vi "MGCC_visualization_phasetwo_v2.vi"() -> ()   [LabVIEW 2016]
uses:
  Black start/Sub-VIs/MGCC_BlkStart_Globals.vi
  MGCC_FntStaMach_gobal.vi
  Resynchronization/MGCC_Resync_global.vi
  Communication/Global communication output.vi
  Communication/Global communication.vi
  <vilib>/imath/engines/lvmath2/RunTimeEngine/IndexRead/NIMS M($,S).vi
  <instcachedir>/0/NIMS M($,S)_3E5749BBB62E49528D4765A77F1F6D98.lvgen/NIMS M($,S)_3E5749BBB62E49528D4765A77F1F6D98_002.vi
  <vilib>/imath/engines/lvmath2/RunTimeEngine/BuiltInFunctions/length/NIMS_length(GV).vi
  <instcachedir>/0/NIMS_length(GV)_08A3D13377FD4E4B96F5795FBF3698FA.lvgen/NIMS_length(GV)_08A3D13377FD4E4B96F5795FBF3698FA_002.vi
  <vilib>/imathl/engines/lvmath/Functions/Error Handling/Create Error.vi
  <vilib>/imath/engines/lvmath2/RunTimeEngine/RangeToken/NIMS_Range_R3 - Integer.vi
  <instcachedir>/0/NIMS_Range_R3 - Integer_A435E2FF893B4C718FD5055FE39FE2F6.lvgen/NIMS_Range_R3 - Integer_A435E2FF893B4C718FD5055FE39FE2F6_000.vi
  <vilib>/imath/engines/lvmath2/RunTimeEngine/CommandStatement/MC_CommandStatement_break.vi
  <vilib>/imath/engines/lvmath2/RunTimeEngine/IndexReplace/NIMS M(S,S)=S.vi
  <instcachedir>/0/NIMS M(S,S)=S_98E40400474E4398B113AE20298B4F82.lvgen/NIMS M(S,S)=S_98E40400474E4398B113AE20298B4F82_002.vi
  <instcachedir>/0/NIMS M($,S)_3E5749BBB62E49528D4765A77F1F6D98.lvgen/NIMS M($,S)_3E5749BBB62E49528D4765A77F1F6D98_000.vi
  <instcachedir>/0/NIMS_length(GV)_08A3D13377FD4E4B96F5795FBF3698FA.lvgen/NIMS_length(GV)_08A3D13377FD4E4B96F5795FBF3698FA_000.vi
  <vilib>/imath/engines/lvmath2/RunTimeEngine/IndexRead/NIMS M(S,$).vi
  <instcachedir>/0/NIMS M(S,$)_F24F360562DE41D8BE234322A2E15C65.lvgen/NIMS M(S,$)_F24F360562DE41D8BE234322A2E15C65_000.vi
  <vilib>/imath/engines/lvmath2/RunTimeEngine/IndexRead/NIMS M(S,S).vi
  <instcachedir>/0/NIMS M(S,S)_AC51E74150A542F7991B9634C66F3096.lvgen/NIMS M(S,S)_AC51E74150A542F7991B9634C66F3096_000.vi
  <instcachedir>/0/NIMS M(S,S)=S_98E40400474E4398B113AE20298B4F82.lvgen/NIMS M(S,S)=S_98E40400474E4398B113AE20298B4F82_000.vi
  <vilib>/imath/engines/lvmath2/RunTimeEngine/BuiltInFunctions/is_empty/NIMS_is_empty(GM).vi
  <instcachedir>/0/NIMS_is_empty(GM)_AF8F13F4B7FD436CB1855477E2504B8A.lvgen/NIMS_is_empty(GM)_AF8F13F4B7FD436CB1855477E2504B8A_004.vi
  <vilib>/imath/engines/lvmath2/RunTimeEngine/IndexRead/NIMS M(R2,S).vi
  <instcachedir>/0/NIMS M(R2,S)_56813DCFDD5A484292D2195AF15D2BF5.lvgen/NIMS M(R2,S)_56813DCFDD5A484292D2195AF15D2BF5_000.vi
  <vilib>/imath/engines/lvmath2/RunTimeSupport/NIMS_Error if Not Equal.vi
  <instcachedir>/0/NIMS_Error if Not Equal_43252A79AD05436189442EC0C5E5AB8A.lvgen/NIMS_Error if Not Equal_43252A79AD05436189442EC0C5E5AB8A_000.vi
  <vilib>/imath/engines/lvmath2/RunTimeEngine/ErrorHandling/NIMS_Create Error From Enums.vi
  <vilib>/imath/engines/lvmath2/RunTimeEngine/NodeEndStatement/NIMS_NodeEndStatement_Output.vi
  <instcachedir>/0/NIMS_NodeEndStatement_Output_53EC0D466D134D7ABD903AC30B43404B.lvgen/NIMS_NodeEndStatement_Output_53EC0D466D134D7ABD903AC30B43404B_010.vi
  <vilib>/imath/engines/lvmath2/RunTimeEngine/ErrorHandling/NIMS_Finalize Error.vi
  <vilib>/imath/engines/lvmath2/RunTimeEngine/BuiltInFunctions/findnz/NIMS_[1o]_findnz(GRowV).vi
  <instcachedir>/0/NIMS_[1o]_findnz(GRowV)_1AF74843B4874134ADE908C0A4A72F3C.lvgen/NIMS_[1o]_findnz(GRowV)_1AF74843B4874134ADE908C0A4A72F3C_000.vi
  <vilib>/imath/engines/lvmath2/RunTimeEngine/BuiltInFunctions/is_empty/NIMS_is_empty(GV).vi
  <instcachedir>/0/NIMS_is_empty(GV)_FC7E7C3D9544432CB6AA2416ADCF6D56.lvgen/NIMS_is_empty(GV)_FC7E7C3D9544432CB6AA2416ADCF6D56_000.vi
  <vilib>/imath/engines/lvmath2/RunTimeEngine/IndexReplace/NIMS V(S)=S.vi
  <instcachedir>/0/NIMS V(S)=S_57E16554CB8B4B90AAB163894F717546.lvgen/NIMS V(S)=S_57E16554CB8B4B90AAB163894F717546_003.vi
  <vilib>/imath/engines/lvmath2/RunTimeEngine/IndexReplace/NIMS V(S)=V.vi
  <instcachedir>/0/NIMS V(S)=V_623363232DF04CF88CEE4AC156064DF2.lvgen/NIMS V(S)=V_623363232DF04CF88CEE4AC156064DF2_000.vi
  <instcachedir>/0/NIMS_NodeEndStatement_Output_53EC0D466D134D7ABD903AC30B43404B.lvgen/NIMS_NodeEndStatement_Output_53EC0D466D134D7ABD903AC30B43404B_004.vi
  <vilib>/imath/engines/lvmath2/RunTimeEngine/IndexRead/NIMS V(S).vi
  <instcachedir>/0/NIMS V(S)_0488751826AF41519A22953C041130DC.lvgen/NIMS V(S)_0488751826AF41519A22953C041130DC_000.vi
  <instcachedir>/0/NIMS V(S)=S_57E16554CB8B4B90AAB163894F717546.lvgen/NIMS V(S)=S_57E16554CB8B4B90AAB163894F717546_000.vi
  <instcachedir>/0/NIMS_NodeEndStatement_Output_53EC0D466D134D7ABD903AC30B43404B.lvgen/NIMS_NodeEndStatement_Output_53EC0D466D134D7ABD903AC30B43404B_005.vi
  State Estimation/Sub-VIs/MGCC_StaEst_global.vi
  Planned Islanding(Mark)/Sub VIs/MGCC_PlanISD_Global.vi
panel:
  in  "planned ISD 29":bool
  in  "planned ISD1":bool
  in  "LC2_reboot":bool
  in  "LC1_reboot":bool
  out "StaEst_An":dbl[][][](array[numeric])
  out "StaEst_Vn":dbl[][][](array[numeric])
  out "Overall MG states":string
  out "L13 line 3":u32(colorbox)
  out "?":bool
  in  "?":dbl(slide) scale=0.0..2.0
  out "LC1 state":string
  out "LC2 state":string
  in  "BKS cmd 2":bool=TRUE
  out "error out":errorcluster
  out "SW 2":u32(colorbox)
  out "G 1":u32(colorbox)
  out "L8":u32(colorbox)
  out "L7 line 2":u32(colorbox)
  out "L6 line 5":u32(colorbox)
  out "L6 line 1":u32(colorbox)
  out "SW 8":u32(colorbox)
  out "SW 8 off":u32(colorbox)
  out "I 8":dbl format="%#.4f"
  out "L6":u32(colorbox)
  out "Communication":bool
  out "Resynchronization":bool
  out "Active power control":bool
  out "Reactive power control":bool
  out "SOC1":dbl=0.5979085480424442 format="%#_4f"
  out "Output":dbl=-9.999999999999723e-06 format="%#_4f"
  in  "PV Mode":bool
  out "Output 3":dbl=0.40429047942961227 format="%#_4f"
  out "Communication 2":bool
  out "Resynchronization 2":bool
  out "Active power control 2":bool
  out "Reactive power control 2":bool
  out "SOC 2":dbl=0.5 format="%#_4f"
  out "Output 2":dbl format="%#_4f"
  out "SW 6":u32(colorbox)
  out "SW 6 off":u32(colorbox)
  out "SW 7":u32(colorbox)
  out "SW 7 off":u32(colorbox)
  out "SW 4":u32(colorbox)
  out "SW 4 off":u32(colorbox)
  out "SW 5":u32(colorbox)
  out "SW 5 off":u32(colorbox)
  out "SW 1":u32(colorbox)
  out "SW 1 off":u32(colorbox)
  out "SW 2 off":u32(colorbox)
  out "SW 3":u32(colorbox)
  out "SW 3 off":u32(colorbox)
  out "I 7":dbl format="%#.4f"
  out "I 3":dbl format="%#.4f"
  out "I 4":dbl format="%#.4f"
  out "I 2":dbl format="%#.4f"
  out "I 6":dbl format="%#.4f"
  out "I 5":dbl format="%#.4f"
  out "I 1":dbl format="%#.4f"
  out "Model Mgmt.":bool
  out "PV Forecasting":bool
  out "Load Forecasting":bool
  out "PQ Balance":bool
  out "Black Start":bool
  out "Data Logging":bool
  out "Communication":bool
  out "State Estimation":bool
  out "Energy Mgmt.":bool
  out "G1 state":string
  in  "Stop":bool
  in  "RESET":bool
  in  "G1":bool
  in  "Ready for STD":bool
  in  "Recon cmd":bool
  in  "BKS cmd":bool=TRUE
  in  "Power Tabs":T1(tab)
  out "Loads Power 6":dbl(graph)
  out "Loads Power 7":dbl(graph)
  out "Loads Power 8":dbl(graph)
  out "Loads Power 9":dbl(graph)
  out "Loads Power 10":dbl(graph)
  out "Loads Power 11":dbl(graph)
  out "Loads Power 12":dbl(graph)
  out "Loads Power 13":dbl(graph)
  in  "Voltage Tabs":T1(tab)
  out "Voltage 6":dbl(graph)
  out "Voltage 7":dbl(graph)
  out "Voltage 8":dbl(graph)
  out "Voltage 9":dbl(graph)
  out "Voltage 10":dbl(graph)
  out "Voltage 11":dbl(graph)
  out "Voltage 12":dbl(graph)
  out "Voltage 13":dbl(graph)
  out "Frequency":T2(graph)
  out "Sources Power":T3(graph)
  out "L11 line 2":u32(colorbox)
  out "L11 line 1":u32(colorbox)
  out "L10 line 2":u32(colorbox)
  out "L12 line 2":u32(colorbox)
  out "G1 line 1":u32(colorbox)
  out "L8 line 2":u32(colorbox)
  out "L8 line 1":u32(colorbox)
  out "L13 line 1":u32(colorbox)
  out "PV line 1":u32(colorbox)
  out "B1 line 1":u32(colorbox)
  out "L13 line 2":u32(colorbox)
  out "B2":bool
  out "SOC Tank 2":dbl(slide) scale=0.0..1.0
  out "PV1":bool
  out "B1":bool
  out "SOC Tank1":dbl(slide) scale=0.0..1.0
  out "PV1 irr Tank":dbl(slide) scale=0.0..2.0
  out "L9 line1":u32(colorbox)
  out "B2 line 1":u32(colorbox)
  out "L9 line 2":u32(colorbox)
  out "L6 line 4":u32(colorbox)
  out "L9":u32(colorbox)
  out "L7":u32(colorbox)
  out "L7 line 1":u32(colorbox)
  out "L8 line 3":u32(colorbox)
  out "L13":u32(colorbox)
  out "L12":u32(colorbox)
  out "L12 line 1":u32(colorbox)
  out "L10 line 1":u32(colorbox)
  out "L11":u32(colorbox)
  out "L10":u32(colorbox)
  out "L6 line 2":u32(colorbox)
  out "L6 line 3":u32(colorbox)
  out "L8 line 4":u32(colorbox)
  out "Gen4 Tank 2":dbl(slide) scale=0.0..1.0
  # "Opal-RT HIL Test Bed Controller"
  # "G5"
  # "SW8"
  # "SW5"
  # "SW1"
  # "SW6"
  # "L6"
  # "L10"
  # "L11"
  # "Local Controller 1"
  # "PV"
  # "BESS1 & PV"
  # "SW2"
  # "SW4"
  # "L7"
  # "L12"
  # "-Manual"
  # "-Profile"
  # "SW7"
  # "SW3"
  # "Local Controller 2"
  # "L8"
  # "Central Controller"
  # "L9"
  # "L13"
  # "BESS2"
  # "Gen4"
  # "BESS1"
  # "PV3"
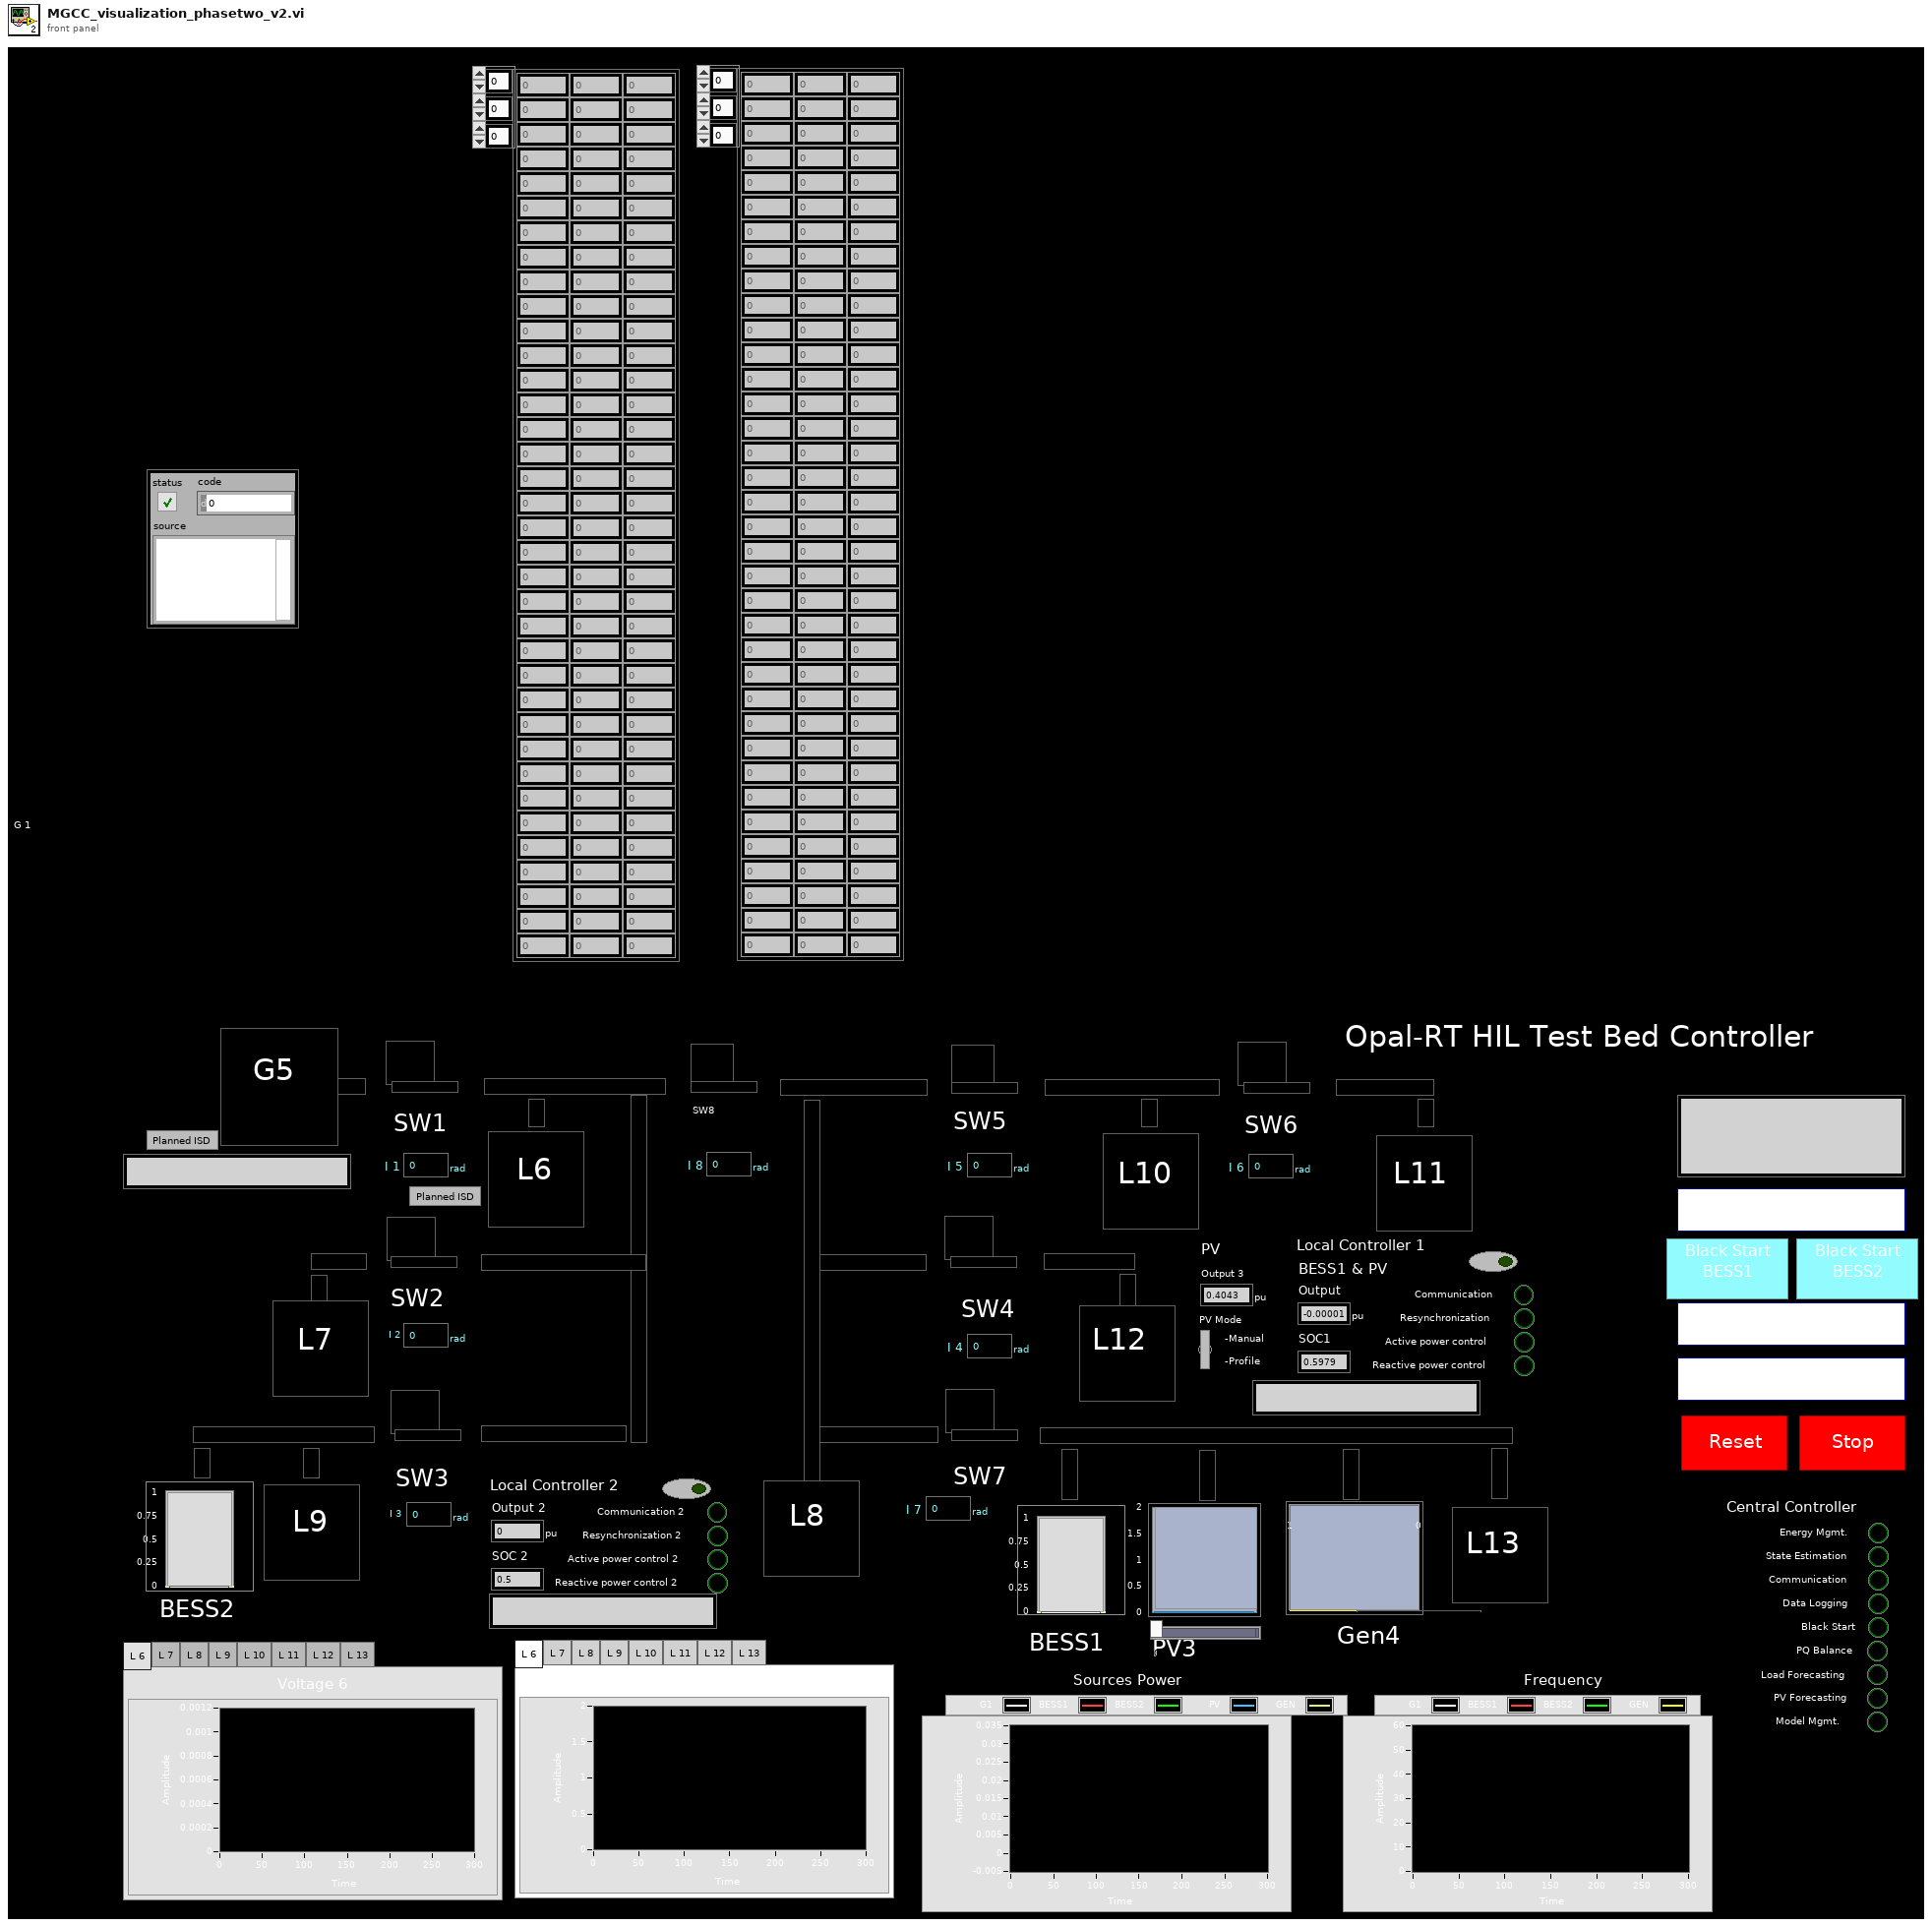
[diagram p1: front panel]
types:
  T1 = enum32{"L 6", "L 7", "L 8", "L 9", "L 10", "L 11", "L 12", "L 13"}
  T2 = cluster{"Numeric":dbl, "Numeric":dbl, "Numeric":dbl, "Numeric 2":dbl}
  T3 = cluster{"Numeric":dbl, "Numeric":dbl, "Numeric":dbl, "Numeric":dbl, "Numeric":dbl}
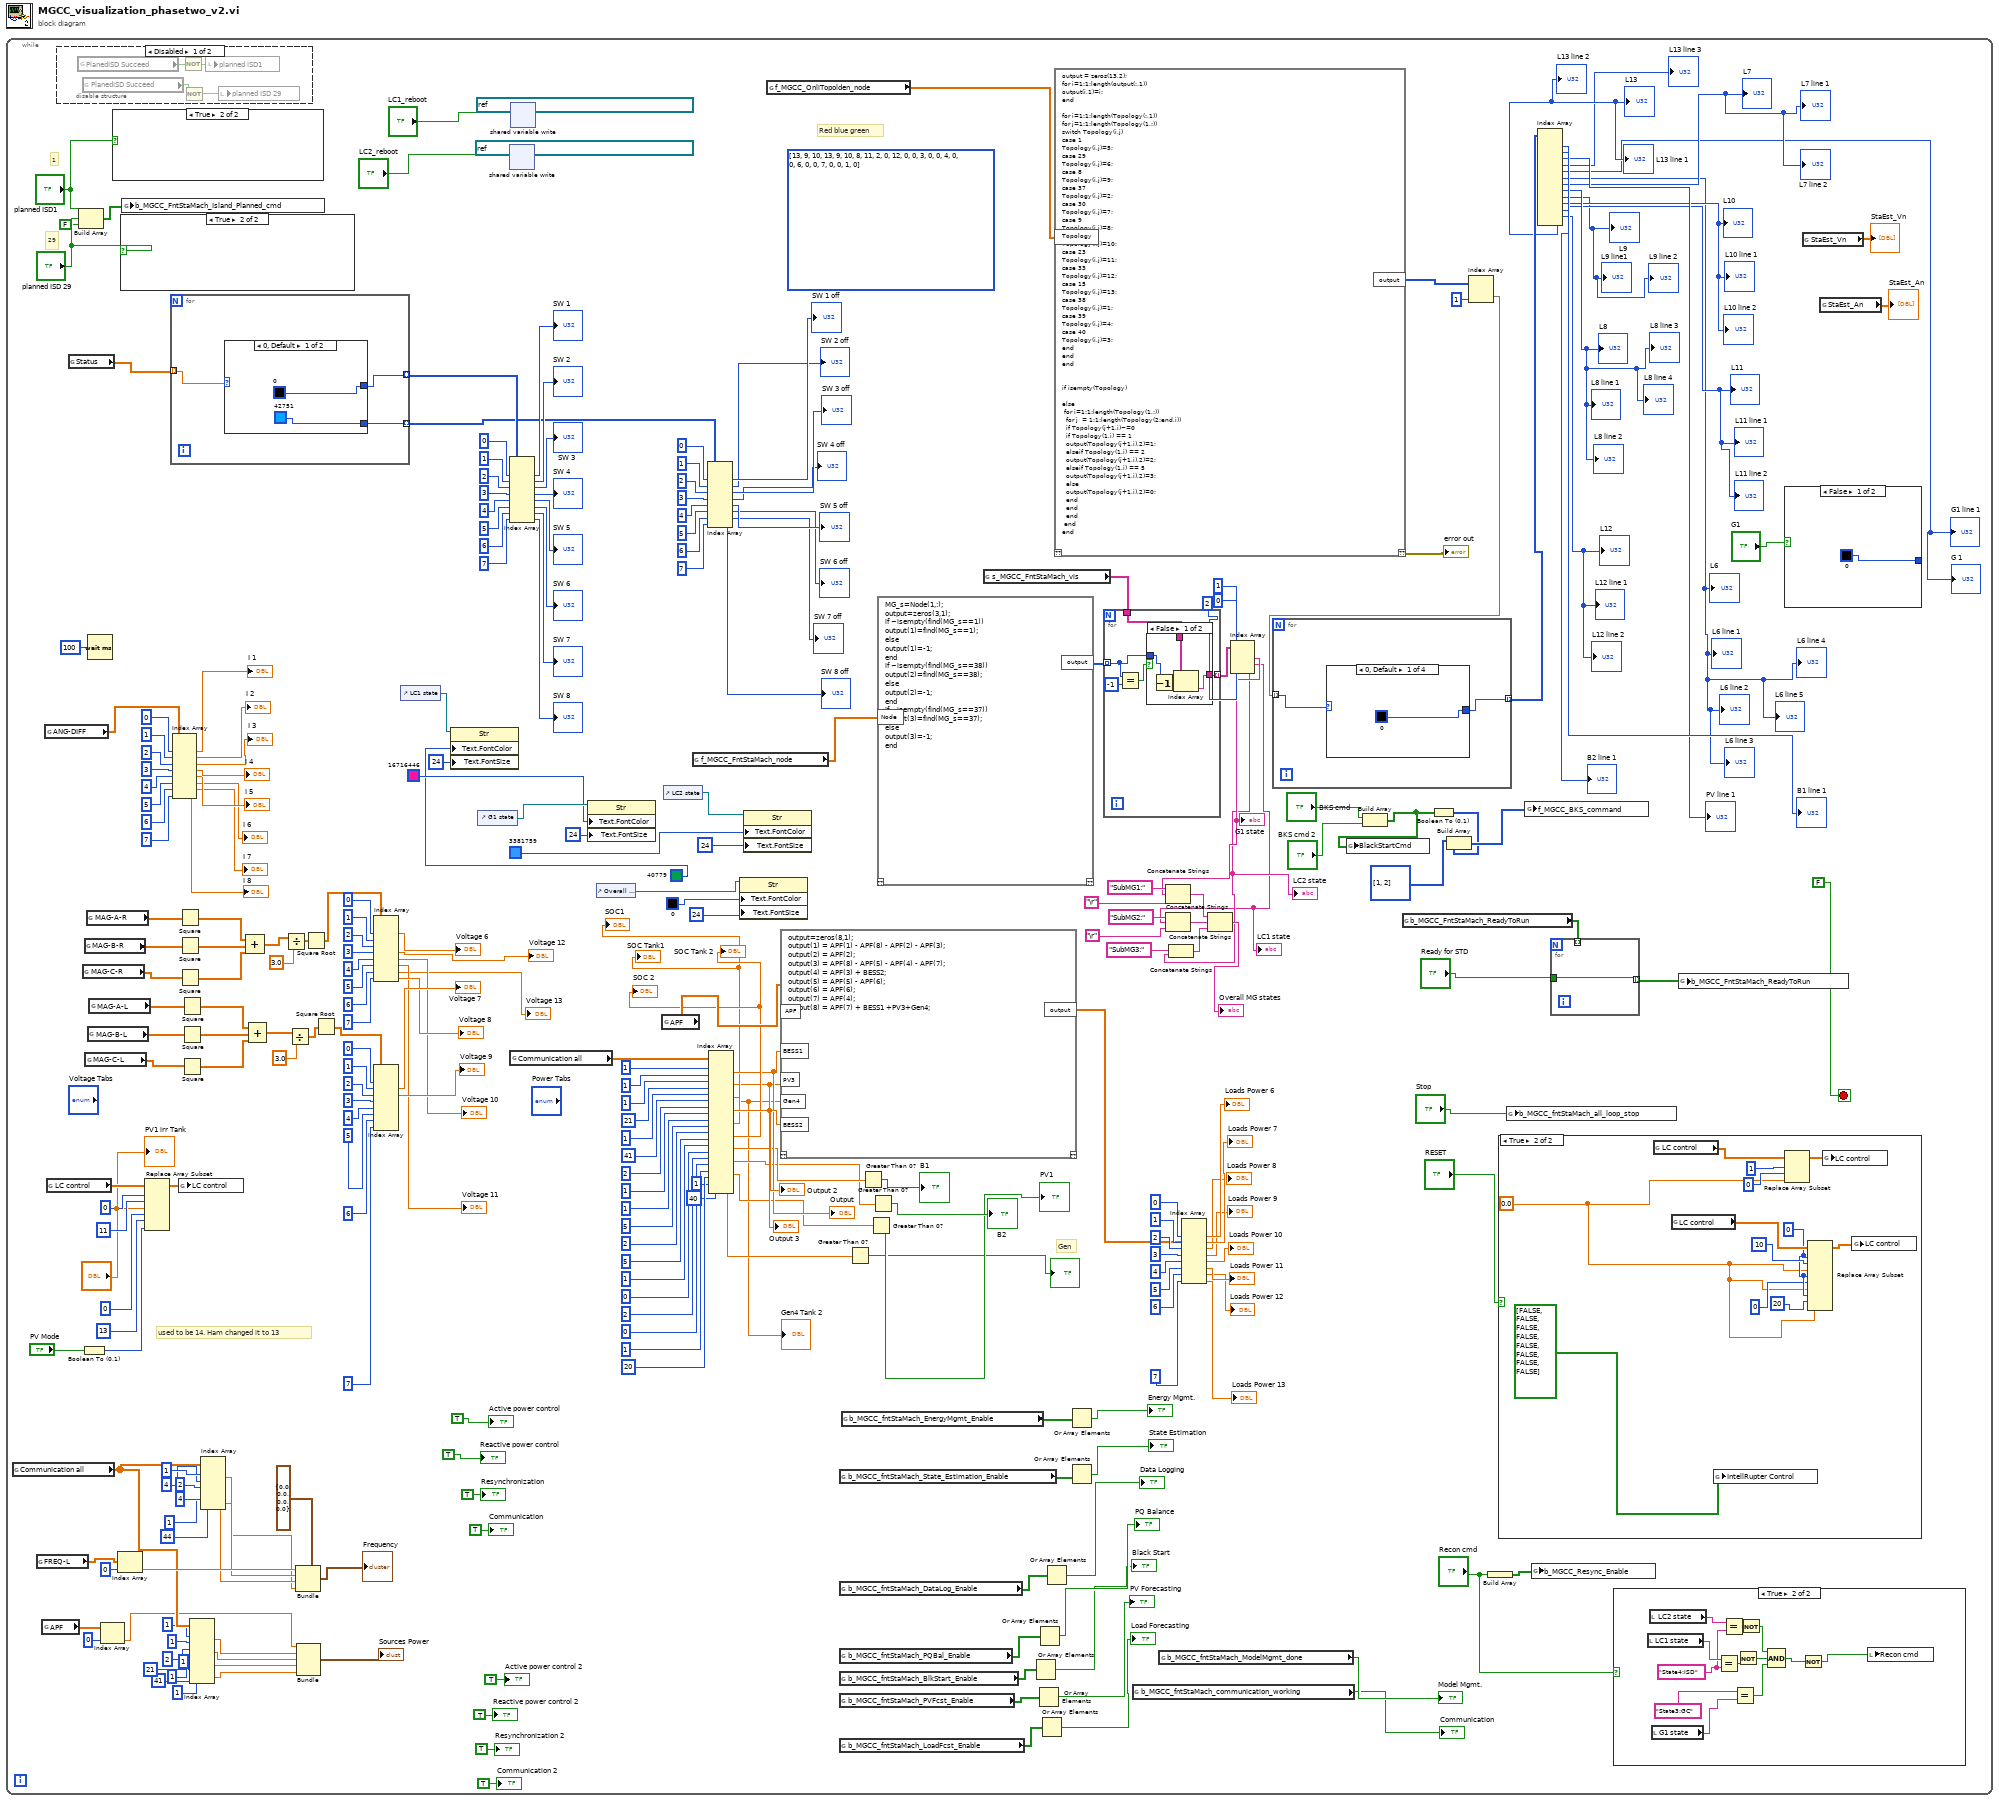
[diagram p0: block diagram]
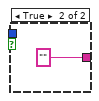
[diagram p7: hidden frame]
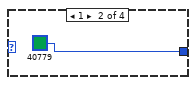
[diagram p8: hidden frame]
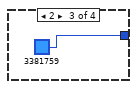
[diagram p9: hidden frame]
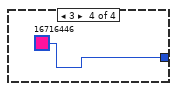
[diagram p10: hidden frame]
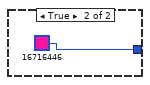
[diagram p11: hidden frame]
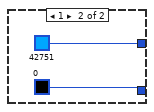
[diagram p12: hidden frame]
diagram:
  n1 = while {
    stop <- FALSE stop-if-true
    (unwired) i32[][] [[13, 9, 10], [13, 9, 10], [8, 11, 2], [0, 12, 0], [0, 3, 0], [0, 4, 0], [0, 6, 0], [0, 7, 0], [0, 1, 0]]
    # "1"
    # "29"
    # "used to be 14. Ham changed it to 13"
    # "Gen"
    # "Red blue green"
    # "9 10: bESS\n11 12: PV gen\n13: g1\n1 to 8: load"
    n2 = global read "Global communication.vi" "Communication all"() -> (w94:dbl[][])
    n3 = global read "Global communication.vi" "FREQ-L"() -> (w99:dbl[])
    n4 = global read "Global communication.vi" "APF"() -> (w87:dbl[])
    n5 = global read "Global communication.vi" "ANG-DIFF"() -> (w206:dbl[])
    n6 = global read "Global communication.vi" "LC control"() -> (w116:dbl[][])
    n7 = disable-structure shown="Disabled" {
      frame Disabled {
        n8 = global read "MGCC_PlanISD_Global.vi" "PlanedISD Succeed"() -> (w292:bool)
        n9 = global read "MGCC_PlanISD_Global.vi" "PlanedISD Succeed"() -> (w290:bool)
        n10 = Not(x=w292) -> (.not. x?=w293:bool)
        n11 = Not(x=w290) -> (.not. x?=w291:bool)
        n12 = local write "planned ISD1"(w293) -> ()
        n13 = local write "planned ISD 29"(w291) -> ()
      }
      frame Enabled {
      }
    }
    n14 = global read "Global communication.vi" "Status"() -> (w289:dbl[])
    n15 = Build Array("planned ISD1", "planned ISD 29", FALSE ("element")) -> (w4:bool[])
    n16 = Boolean To (0,1)(Boolean="PV Mode") -> (0, 1=w104:i16)
    n17 = global read "Global communication.vi" "MAG-C-R"() -> (w189:dbl[])
    n18 = global read "Global communication.vi" "MAG-B-R"() -> (w190:dbl[])
    n19 = global read "Global communication.vi" "MAG-C-L"() -> (w195:dbl[])
    n20 = global read "Global communication.vi" "MAG-A-R"() -> (w191:dbl[])
    n21 = Wait (ms)(milliseconds to wait=u32 100) -> ()  [unwired: 1 out]
    n22 = global read "Global communication.vi" "MAG-B-L"() -> (w196:dbl[])
    n23 = global read "Global communication.vi" "MAG-A-L"() -> (w197:dbl[])
    n24 = Index Array(array=w87, index=0) -> (element=w85:dbl)
    n25 = case shown="True" "planned ISD1" {
      frame False {
      }
      frame True {
      }
    }
    n26 = Index Array(array=w99, index=0) -> (element=w97:dbl)
    n27 = case shown="True" "planned ISD 29" {
      frame False {
      }
      frame True {
      }
    }
    n28 = global write "MGCC_FntStaMach_gobal.vi" "b_MGCC_FntStaMach_Island_Planned_cmd"(w4) -> ()
    n29 = Replace Array Subset(array=w116, new element #1="?", index (row) #1=0 ("index (row)"), index (col) #1=11 ("disabled index (col)"), new element #2=w104, index (row) #2=0 ("index (row)"), index (col) #2=13 ("disabled index (col)")) -> (w115:dbl[][])
    n30 = for {
      tunnel: w289 -> [w2198] mode=indexing
      tunnel: [w2197] -> w288 mode=indexing
      tunnel: [w2196] -> w263 mode=indexing
      n31 = case shown="0, Default" w2198 {
        tunnel: [u32 0 ("Color Box 17") u32 42751 ("Color Box 17")] -> w2197
        tunnel: [u32 42751 ("Color Box 17") u32 0 ("Color Box 17")] -> w2196
        frame 0, Default {
        }
        frame 1 {
        }
      }
    }
    n32 = Index Array(array=w206, index #1=0 ("index"), index #2=1 ("index"), index #3=2 ("index"), index #4=3 ("index"), index #5=4 ("index"), index #6=5 ("index"), index #7=6 ("index"), index #8=7 ("index")) -> (element #1=→"I 1":dbl, element #2=→"I 2":dbl, element #3=→"I 3":dbl, element #4=→"I 4":dbl, element #5=→"I 5":dbl, element #6=→"I 6":dbl, element #7=→"I 7":dbl, element #8=→"I 8":dbl)
    n33 = Square(x=w191) -> (x^2=w188:dbl[])
    n34 = Square(x=w190) -> (x^2=w187:dbl[])
    n35 = Square(x=w189) -> (x^2=w186:dbl[])
    n36 = global write "Global communication.vi" "LC control"(w115) -> ()
    n37 = Square(x=w197) -> (x^2=w194:dbl[])
    n38 = Square(x=w196) -> (x^2=w193:dbl[])
    n39 = Square(x=w195) -> (x^2=w192:dbl[])
    n40 = Index Array(array=w94, index (row) #1=1 ("index (row)"), index (col) #1=1 ("disabled index (col)"), index (row) #2=2 ("index (row)"), index (col) #2=1 ("disabled index (col)"), index (row) #3=1 ("index (row)"), index (col) #3=21 ("disabled index (col)"), index (row) #4=1 ("index (row)"), index (col) #4=41 ("disabled index (col)")) -> (element #1=w89:dbl, element #2=w88:dbl, element #3=w18:dbl, element #4=w17:dbl)
    n41 = Index Array(array=w94, index (row) #1=1 ("index (row)"), index (col) #1=4 ("disabled index (col)"), index (row) #2=2 ("index (row)"), index (col) #2=4 ("disabled index (col)"), index (row) #3=1 ("index (row)"), index (col) #3=44 ("disabled index (col)")) -> (element #1=w96:dbl, element #2=w95:dbl, element #3=w14:dbl)
    n42 = Compound Arithmetic op=ADD(w188, w187, w186) -> (w11:dbl[])
    n43 = Compound Arithmetic op=ADD(w194, w193, w192) -> (w8:dbl[])
    n44 = Divide(x=w11, y=3.0) -> (x/y=w12:dbl[])
    n45 = Divide(x=w8, y=3.0) -> (x/y=w7:dbl[])
    n46 = Bundle(cluster=T2 {"Numeric"=0.0, "Numeric"=0.0, "Numeric"=0.0, "Numeric 2"=0.0}, "Numeric"=w97, "Numeric"=w96, "Numeric"=w95, "Numeric 2"=w14) -> (→"Frequency":T2)
    n47 = Bundle("Numeric"=w85, "Numeric"=w89, "Numeric"=w88, "Numeric"=w18, "Numeric"=w17) -> (→"Sources Power":T3)  [unwired: 1 in]
    n48 = Square Root(x=w12) -> (sqrt(x)=w169:dbl[])
    n49 = Square Root(x=w7) -> (sqrt(x)=w168:dbl[])
    n50 = Index Array(array=w169, index #1=0 ("index"), index #2=1 ("index"), index #3=2 ("index"), index #4=3 ("index"), index #5=4 ("index"), index #6=5 ("index"), index #7=6 ("index"), index #8=7 ("index")) -> (element #1=→"Voltage 6":dbl, element #4=→"Voltage 12":dbl, element #5=→"Voltage 10":dbl, element #6=→"Voltage 11":dbl, element #7=→"Voltage 13":dbl, element #8=→"Voltage 8":dbl)  [unwired: 2 out]
    n51 = Index Array(array=w168, index #1=0 ("index"), index #2=1 ("index"), index #3=2 ("index"), index #4=3 ("index"), index #5=4 ("index"), index #6=5 ("index"), index #7=6 ("index"), index #8=7 ("index")) -> (element #2=→"Voltage 7":dbl, element #3=→"Voltage 9":dbl)  [unwired: 6 out]
    n52 = control-ref of="LC1 state"() -> (w219:refnum<vi>)
    n53 = property on="Property Node" class="Str"(reference=w219, "Text.FontColor"=u32 40779 ("Color Box 17"), "Text.FontSize"=u32 24 ("Text.Font:Size")) -> ()  [unwired: 1 in, 2 out]
    n54 = control-ref of="G1 state"() -> (w223:refnum<vi>)
    n55 = shared-variable-write(refnum<k21> "ni.var.psp://LC2/Untitled Library 2/LC2_reboot" ("shared variable refnum in"), "LC2_reboot") -> ()  [unwired: 1 in, 2 out]
    n56 = Index Array(array=w288, index #1=0 ("index"), index #2=1 ("index"), index #3=2 ("index"), index #4=3 ("index"), index #5=4 ("index"), index #6=5 ("index"), index #7=6 ("index"), index #8=7 ("index")) -> (element #1=→"SW 1":u32, element #2=→"SW 2":u32, element #3=→"SW 3":u32, element #4=→"SW 4":u32, element #5=→"SW 5":u32, element #6=→"SW 6":u32, element #7=→"SW 7":u32, element #8=→"SW 8":u32)
    n57 = global read "Global communication.vi" "Communication all"() -> (w141:dbl[][])
    n58 = shared-variable-write(refnum<k21> "ni.var.psp://LC1/Untitled Library 1/LC1_reboot" ("shared variable refnum in"), "LC1_reboot") -> ()  [unwired: 1 in, 2 out]
    n59 = property on="Property Node" class="Str"(reference=w223, "Text.FontColor"=u32 16716446 ("Color Box 17"), "Text.FontSize"=u32 24 ("Text.Font:Size")) -> ()  [unwired: 1 in, 2 out]
    n60 = control-ref of="Overall MG states"() -> (w29:refnum<vi>)
    n61 = global read "Global communication.vi" "APF"() -> (w159:dbl[])
    n62 = control-ref of="LC2 state"() -> (w218:refnum<vi>)
    n63 = global read "MGCC_FntStaMach_gobal.vi" "f_MGCC_FntStaMach_node"() -> (w230:dbl[])
    n64 = Index Array(array=w263, index #1=0 ("index"), index #2=1 ("index"), index #3=2 ("index"), index #4=3 ("index"), index #5=4 ("index"), index #6=5 ("index"), index #7=6 ("index"), index #8=7 ("index")) -> (element #1=→"SW 1 off":u32, element #2=→"SW 2 off":u32, element #3=→"SW 3 off":u32, element #4=→"SW 4 off":u32, element #5=→"SW 5 off":u32, element #6=→"SW 6 off":u32, element #7=→"SW 7 off":u32, element #8=→"SW 8 off":u32)
    n65 = Index Array(array=w141, index (row) #1=1 ("index (row)"), index (col) #1=1 ("disabled index (col)"), index (row) #2=1 ("index (row)"), index (col) #2=21 ("disabled index (col)"), index (row) #3=1 ("index (row)"), index (col) #3=41 ("disabled index (col)"), index (row) #4=2 ("index (row)"), index (col) #4=1 ("disabled index (col)"), index (row) #5=1 ("index (row)"), index (col) #5=5 ("disabled index (col)"), index (row) #6=2 ("index (row)"), index (col) #6=5 ("disabled index (col)"), index (row) #7=1 ("index (row)"), index (col) #7=0 ("disabled index (col)"), index (row) #8=2 ("index (row)"), index (col) #8=0 ("disabled index (col)"), index (row) #9=1 ("index (row)"), index (col) #9=20 ("disabled index (col)"), index (row) #10=1 ("index (row)"), index (col) #10=40 ("disabled index (col)")) -> (element #1=w127:dbl, element #2=w125:dbl, element #3=w42:dbl, element #4=w129:dbl, element #5=→"SOC Tank1" →"SOC1":dbl, element #6=→"SOC 2" →"SOC Tank 2":dbl, element #7=w120:dbl, element #8=w118:dbl, element #9=w109:dbl, element #10=w45:dbl)
    "Output 2" <- w129
    "Output" <- w127
    "Output 3" <- w125
    "Gen4 Tank 2" <- w42
    n66 = property on="Property Node" class="Str"(reference=w29, "Text.FontColor"=u32 0 ("Color Box 17"), "Text.FontSize"=u32 24 ("Text.Font:Size")) -> ()  [unwired: 1 in, 2 out]
    n67 = property on="Property Node" class="Str"(reference=w218, "Text.FontColor"=u32 3381759 ("Color Box 17"), "Text.FontSize"=u32 24 ("Text.Font:Size")) -> ()  [unwired: 1 in, 2 out]
    n68 = global read "MGCC_FntStaMach_gobal.vi" "f_MGCC_OnliTopolden_node"() -> (w246:dbl[][])
    n69 = mathscript code="output=zeros(8,1);\noutput(1) = APF(1) - APF(8) - APF(2) - APF(3);\noutput(2) = APF(2);\noutput(3) = APF(8) - APF(5) - APF(4) - APF(7);\noutput(4) = APF(3) + BESS2;\noutput(5) = APF(5) - APF(6);\noutput(6) = APF(6);\noutput(7) = APF(4);\noutput(8) = APF(7) + BESS1 +PV3+Gen4;"("APF"=w159, "BESS1"=w127, "PV3"=w125, "Gen4"=w42, "BESS2"=w129) -> ("output"=w150:dbl[])  [unwired: 1 in, 1 out]
    n70 = global read "MGCC_FntStaMach_gobal.vi" "b_MGCC_fntStaMach_State_Estimation_Enable"() -> (w73:bool[])
    n71 = global read "MGCC_FntStaMach_gobal.vi" "b_MGCC_fntStaMach_DataLog_Enable"() -> (w71:bool[])
    n72 = global read "MGCC_FntStaMach_gobal.vi" "b_MGCC_fntStaMach_PQBal_Enable"() -> (w69:bool[])
    n73 = global read "MGCC_FntStaMach_gobal.vi" "b_MGCC_fntStaMach_BlkStart_Enable"() -> (w67:bool[])
    n74 = global read "MGCC_FntStaMach_gobal.vi" "b_MGCC_fntStaMach_PVFcst_Enable"() -> (w65:bool[])
    n75 = global read "MGCC_FntStaMach_gobal.vi" "b_MGCC_fntStaMach_LoadFcst_Enable"() -> (w63:bool[])
    n76 = global read "MGCC_FntStaMach_gobal.vi" "b_MGCC_fntStaMach_EnergyMgmt_Enable"() -> (w75:bool[])
    n77 = Greater Than 0?(x=w45) -> (x > 0?=→"?":bool)
    n78 = Greater Than 0?(x=w120) -> (x > 0?=→"B1":bool)
    n79 = Greater Than 0?(x=w109) -> (x > 0?=→"PV1":bool)
    n80 = Greater Than 0?(x=w118) -> (x > 0?=→"B2":bool)
    n81 = mathscript code="MG_s=Node(1,:);\noutput=zeros(3,1);\nif ~isempty(find(MG_s==1))\noutput(1)=find(MG_s==1);\nelse\noutput(1)=-1;\nend\nif ~isempty(find(MG_s==38))\noutput(2)=find(MG_s==38);\nelse\noutput(2)=-1;\nend\nif ~isempty(find(MG_s==37))\noutput(3)=find(MG_s==37);\nelse\noutput(3)=-1;\nend"("Node"=w230) -> ("output"=w229:i32[])  [unwired: 1 in, 1 out]
    n82 = global read "MGCC_FntStaMach_gobal.vi" "s_MGCC_FntStaMach_vis"() -> (w228:string[])
    n83 = Or Array Elements(Boolean array=w67) -> (logical OR=→"Black Start":bool)
    n84 = Or Array Elements(Boolean array=w65) -> (logical OR=→"PV Forecasting":bool)
    n85 = Or Array Elements(Boolean array=w69) -> (logical OR=→"PQ Balance":bool)
    n86 = Or Array Elements(Boolean array=w63) -> (logical OR=→"Load Forecasting":bool)
    n87 = Or Array Elements(Boolean array=w71) -> (logical OR=→"Data Logging":bool)
    n88 = mathscript code="output = zeros(13,2);\nfor i=1:1:length(output(:,1))\noutput(i,1)=i;\nend\n\nfor i=1:1:length(Topology(:,1))\nfor j=1:1:length(Topology(1,:))\nswitch Topology(i,j)\ncase 1\nTopology(i,j)=5;\ncase 29\nTopology(i,j)=6;\ncase 8\nTopology(i,j)=9;\ncase 37\nTopology(i,j)=2;\ncase 30\nTopology(i,j)=7;\ncase 9\nTopology(i,j)=8;\ncase 35\nTopology(i,j)=10;\ncase 23\nTopology(i,j)=11;\ncase 33\nTopology(i,j)=12;\ncase 15\nTopology(i,j)=13;\ncase 38\nTopology(i,j)=1;\ncase 39\nTopology(i,j)=4;\ncase 40\nTopology(i,j)=3;\nend\nend\nend\n\n\nif isempty(Topology)\n\nelse\n for i=1:1:length(Topology(1,:))\n  for j  = 1:1:length(Topology(2:end,i))\n  if Topology(j+1,i)~=0\n  if Topology(1,i) == 1\n  output(Topology(j+1,i),2)=1;\n  elseif Topology(1,i) == 2\n  output(Topology(j+1,i),2)=2;\n  elseif Topology(1,i) == 5\n  output(Topology(j+1,i),2)=3;\n  else\n  output(Topology(j+1,i),2)=0;\n  end\n  end\n  end\n end\nend"("Topology"=w246) -> ("??"=→"error out":errorcluster, "output"=w251:i32[][])  [unwired: 1 in]
    n89 = Or Array Elements(Boolean array=w75) -> (logical OR=→"Energy Mgmt.":bool)
    n90 = Or Array Elements(Boolean array=w73) -> (logical OR=→"State Estimation":bool)
    n91 = for {
      tunnel: w229 -> [w596] mode=indexing
      tunnel: w228 -> [w595]
      tunnel: [w594] -> w227 mode=indexing
      n92 = Equal?(x=w596, y=-1) -> (x = y?=w597:bool)
      n93 = case shown="False" w597 {
        tunnel: [w599 ""] -> w594
        tunnel: w596 -> [w601 _]
        tunnel: w595 -> [w600 _]
        frame False {
          n94 = Decrement(x=w601) -> (x-1=w602:i32)
          n95 = Index Array(array=w600, index=w602) -> (element=w599:string)
        }
        frame True {
        }
      }
    }
    n96 = global read "MGCC_FntStaMach_gobal.vi" "b_MGCC_fntStaMach_communication_working"() -> (→"Communication":bool)
    n97 = global read "MGCC_FntStaMach_gobal.vi" "b_MGCC_fntStaMach_ModelMgmt_done"() -> (→"Model Mgmt.":bool)
    n98 = Index Array(array=w150, index #1=0 ("index"), index #2=1 ("index"), index #3=2 ("index"), index #4=3 ("index"), index #5=4 ("index"), index #6=5 ("index"), index #7=6 ("index"), index #8=7 ("index")) -> (element #1=→"Loads Power 6":dbl, element #2=→"Loads Power 7":dbl, element #3=→"Loads Power 8":dbl, element #4=→"Loads Power 9":dbl, element #5=→"Loads Power 10":dbl, element #6=→"Loads Power 11":dbl, element #7=→"Loads Power 12":dbl, element #8=→"Loads Power 13":dbl)
    n99 = Index Array(array=w227, index #1=0 ("index"), index #2=1 ("index"), index #3=2 ("index")) -> (element #1=w40:string, element #2=w19:string, element #3=w20:string)
    "LC2 state" <- w20
    "LC1 state" <- w19
    "G1 state" <- w40
    n100 = Concatenate Strings("SubMG1:", w40, "\r") -> (w35:string)
    n101 = Concatenate Strings("SubMG2:", w19, "\r") -> (w34:string)
    n102 = Concatenate Strings("SubMG3:", w20) -> (w33:string)
    n103 = Concatenate Strings(w35, w34, w33) -> (→"Overall MG states":string)
    n104 = Build Array("BKS cmd", "BKS cmd 2") -> (w13:bool[])
    n105 = global write "MGCC_BlkStart_Globals.vi" "BlackStartCmd"(w13) -> ()
    n106 = global read "MGCC_FntStaMach_gobal.vi" "b_MGCC_FntStaMach_ReadyToRun"() -> (w59:bool[])
    n107 = Boolean To (0,1)(Boolean=w13) -> (0, 1=w234:i16[])
    n108 = Build Array(i32[] [1, 2], w234) -> (w235:i32[][])
    n109 = Index Array(array=w251, index (col)=1 ("disabled index (col)")) -> (element=w249:i32[])  [unwired: 1 in]
    n110 = for {
      tunnel: w249 -> [w827] mode=indexing
      tunnel: [w826] -> w248 mode=indexing
      n111 = case shown="0, Default" w827 {
        tunnel: [u32 0 ("Color Box 17") u32 40779 ("Color Box 17") u32 3381759 ("Color Box 17") u32 16716446 ("Color Box 17")] -> w826
        frame 0, Default {
        }
        frame 1 {
        }
        frame 2 {
        }
        frame 3 {
        }
      }
    }
    n112 = Build Array("Recon cmd") -> (w6:bool[])
    n113 = case shown="True" "RESET" {
      frame False {
      }
      frame True {
        w307 = 0.0 ("new element/subarray")
        w310 = 0 ("index")
        n114 = global read "Global communication.vi" "LC control"() -> (w316:dbl[][])
        n115 = global read "Global communication.vi" "LC control"() -> (w314:dbl[][])
        n116 = global write "Global communication output.vi" "IntellRupter Control"(bool[] [FALSE, FALSE, FALSE, FALSE, FALSE, FALSE, FALSE, FALSE] ("IntellRupter Control")) -> ()
        n117 = Replace Array Subset(array=w316, new element=w307, index (row)=1 ("index"), index (col)=0 ("index")) -> (w315:dbl[][])
        n118 = Replace Array Subset(array=w314, new element #1=w307, index (row) #1=w310, index (col) #1=10 ("index"), new element #2=w307, index (row) #2=w310, index (col) #2=0 ("index"), new element #3=w307, index (row) #3=w310, index (col) #3=20 ("index")) -> (w313:dbl[][])
        n119 = global write "Global communication.vi" "LC control"(w315) -> ()
        n120 = global write "Global communication.vi" "LC control"(w313) -> ()
      }
    }
    n121 = global write "MGCC_FntStaMach_gobal.vi" "b_MGCC_fntStaMach_all_loop_stop"("Stop") -> ()
    n122 = global write "MGCC_FntStaMach_gobal.vi" "f_MGCC_BKS_command"(w235) -> ()
    n123 = global write "MGCC_Resync_global.vi" "b_MGCC_Resync_Enable"(w6) -> ()
    n124 = Index Array(array=w248) -> (element #1=→"B1 line 1":u32, element #2=→"B2 line 1":u32, element #3=→"PV line 1":u32, element #4=→"L13 line 3":u32, element #5=→"G1 line 1" →"G 1":u32, element #6=→"L6" →"L6 line 2" →"L6 line 1" →"L6 line 3" →"L6 line 4" →"L6 line 5":u32, element #7=→"L7" →"L7 line 1" →"L7 line 2":u32, element #8=→"L8 line 3" →"L8 line 1" →"L8 line 4" →"L8 line 2" →"L8":u32, element #9=→"L9 line1" →"L9" →"L9 line 2":u32, element #10=→"L10 line 2" →"L10 line 1" →"L10":u32, element #11=→"L11" →"L11 line 1" →"L11 line 2":u32, element #12=→"L12 line 1" →"L12 line 2" →"L12":u32, element #13=→"L13 line 1" →"L13" →"L13 line 2":u32)  [unwired: 13 in]
    n125 = for {
      tunnel: w59 -> [_] mode=indexing
      tunnel: "Ready for STD" -> [w318]
      tunnel: [w318] -> w57 mode=indexing
    }
    n126 = case shown="True" "Recon cmd" {
      frame False {
      }
      frame True {
        w303 = "State4:ISD"
        n127 = local read "LC1 state"() -> (w305:string)
        n128 = local read "LC2 state"() -> (w304:string)
        n129 = local read "G1 state"() -> (w302:string)
        n130 = Equal?(x=w305, y=w303) -> (x = y?=w299:bool)
        n131 = Equal?(x=w304, y=w303) -> (x = y?=w300:bool)
        n132 = Equal?(x="State3:GC", y=w302) -> (x = y?=w298:bool)
        n133 = Not(x=w299) -> (.not. x?=w294:bool)
        n134 = Not(x=w300) -> (.not. x?=w295:bool)
        n135 = Compound Arithmetic op=AND(w295, w294, w298) -> (w297:bool)
        n136 = Not(x=w297) -> (.not. x?=w296:bool)
        n137 = local write "Recon cmd"(w296) -> ()
      }
    }
    n138 = global write "MGCC_FntStaMach_gobal.vi" "b_MGCC_FntStaMach_ReadyToRun"(w57) -> ()
    n139 = case shown="False" "G1" {
      tunnel: [u32 0 ("Color Box 17") u32 16716446 ("Color Box 17")] -> _
      frame False {
      }
      frame True {
      }
    }
    n140 = global read "MGCC_StaEst_global.vi" "StaEst_Vn"() -> (→"StaEst_Vn":dbl[][][])
    n141 = global read "MGCC_StaEst_global.vi" "StaEst_An"() -> (→"StaEst_An":dbl[][][])
    "PV1 irr Tank" <- "?"
    "Reactive power control 2" <- TRUE ("Reactive power control 2")
    "Active power control 2" <- TRUE ("Active power control 2")
    "Resynchronization 2" <- TRUE ("Resynchronization 2")
    "Communication 2" <- TRUE ("Communication 2")
    "Reactive power control" <- TRUE ("Reactive power control")
    "Active power control" <- TRUE ("Active power control")
    "Resynchronization" <- TRUE ("Resynchronization")
    "Communication" <- TRUE ("Communication")
  }
